vi "2100_Test_Set State_Measure Resistance_SH3T_Ron_w Config.vi"(0 "Semiconductor Module Context":T7, 1 "Script_Info":T3={"Script Name"="WalkingState", "All_Scripts"=[]}, 4 "Instrument_Pins":T6={"SMU_Pins"=["RF1", "RF2", "RF3", "RF4"], "HSDIO_Pins"=["CLK", "SDA"]}, 5 "Error In":errorcluster, 6 "USID":T4 max=15, 7 "Master_Register_Data_Array_In":T1 {"Address" format="%.0x"}, 8 "current range":dbl format="%#_6p", 9 "current level":dbl=1e-05 format="%#_13p", 10 "Publishable IDs":string[](array[string])=["State00", "State01", "State02", "State04", "State08"], 11 "Reg_Map_and_Bit_Name":T5={"Reg_Map_Bit_Name"="", "Reg_Map"=[["Reg Addr(0x00)", "7", "6", "5", "4", "3", "2", "1", "0"], ["0", "SPARE", "RF3_SH", "RF2_SH", "RF1_SH", "SPARE", "RF3_RFC", "RF2_RFC", "RF1_RFC"], ["1", "SPARE[7:0]", "", "", "", "", "", "", ""], ["2", "VVAR_EN", "LCM_EN", "RFC_SH", "SPARE", "VARACTOR[3:0]", "", "", ""], ["3", "SW_CTRL1_VIRTUAL[7:0]", "", "", "", "", "", "", ""], ["4", "SW_CTRL1_SWAP", "SW_CTRL1_RBSHIFT[2:0]", "", "", "SW_CTRL1_VSID[3:0]", "", "", ""], ["5", "REG_00_VIRTUAL_MASK[7:0]", "", "", "", "", "", "", ""], ["6", "LOCK_STATUS[1:0]", "", "CLK_DITHER", "FUSES_BURNED", "CLK_IDAC_CAL[3:0]", "", "", ""], ["7", "SPARE[2:0]", "", "", "ODFT_TRIM[4:0]", "", "", "", ""], ["8", "SPARE[2:0]", "", "", "HV_TRIM[4:0]", "", "", "", ""], ["9", "TEST_MUX[2:0]", "", "", "SPARE[1:0]", "", "MEMS_BG_TC[1:0]", "", "MEMSCP_RCM"], ["A", "CP_BOOST_OVRD_EN", "SPARE[2:0]", "", "", "PS_OFF_TIMER[1:0]", "", "PS_ON_TIMER[1:0]", ""], ["0", "", "", "", "", "", "", "", ""], ["D", "Reserved[1:0]", "", "WD_HI_EVENT_CNT[5:0]", "", "", "", "", ""], ["E", "VERSION_ID[7:0]", "", "", "", "", "", "", ""], ["F", "Reserved", "COUNT_200_LSB[6:0]", "", "", "", "", "", ""], ["10", "CLK_DIV2_EN", "Spare", "ODFT_EN", "HV_HYST[4:0]", "", "", "", ""], ["0", "", "", "", "", "", "", "", ""], ["12", "SHORT_FUSE", "FUSE_BURN", "STROBE_EN", "VIO_OK", "RTH[1:0]", "", "FUSE_LOAD_MAN_EN", "FUSE_LOAD"], ["13", "RR_ACK_EN", "Reserved", "ACK_POSITION[1:0]", "", "SuBUS_DRIVE_STRENGTH[3:0]", "", "", ""], ["14", "TM_IO_EN", "TM_IO_SEL", "SuBUS_OVS[1:0]", "", "Reserved[3:0]", "", "", ""], ["15", "Reserved[4:0]", "", "", "", "", "SuBUS_VERSION_PRESENT", "SuBUS_VOLTAGE", "SuBUS_FLAVOR_DEF"], ["16", "PROG_STROBE1_DUR[7:0]", "", "", "", "", "", "", ""], ["17", "PROG_STROBE0_DUR[7:0]", "", "", "", "", "", "", ""], ["18", "Reserved[2:0]", "", "", "EFUSE_SINGLE_ADDR_SEL[4:0]", "", "", "", ""], ["19", "POLL_ADR[4:0]", "", "", "", "", "POLL_BC[2:0]", "", ""], ["1A", "SOFTWARE_RESET", "Reserved[6:0]", "", "", "", "", "", ""], ["1B", "Reserved[7:0]", "", "", "", "", "", "", ""], ["1C", "PWR_MODE_1", "PWR_MODE_0", "TRIGGER_MASK[2:0]", "", "", "TRIGGER[2:0]", "", ""], ["1D", "PRODUCT_ID[7:0]", "", "", "", "", "", "", ""], ["1E", "MANUFACTURER_ID_LSB[7:0]", "", "", "", "", "", "", ""], ["1F", "MANUFACTURER_ID_MSB[3:0]", "", "", "", "USID[3:0]", "", "", ""]]}, 12 "R_Guardian":dbl[](array[numeric])) -> (15 "Master_Register_Data_Array_Out":T1 {"Address" format="%.0x"}, 19 "Error Out":errorcluster)   [LabVIEW 2013]
uses:
  Controls/USID.ctl
  <vilib>/NI_TestStand_SemiconductorModule/NI_TestStand_Semiconductor_Module.lvlibp/PinMap/General/SemiconductorModuleContext.ctl
  Controls/Master_Reg_Data_Array.ctl
  Controls/Reg_Address_Data.ctl
  <vilib>/NI_TestStand_SemiconductorModule/NI_TestStand_Semiconductor_Module.lvlibp/PinMap/General/Publish/PublishDataDoubleFunctionalTest.vi
  <vilib>/NI_TestStand_SemiconductorModule/NI_TestStand_Semiconductor_Module.lvlibp
panel:
  out "Publishable IDs 2":string[](array[string])=["State00", "State01", "State02", "State04", "State08"]
  out "Logged_Data":dbl[](array[numeric]) format="%#_6p"
  out "R_Measurements":dbl[](array[numeric]) format="%#_6p"
  in  "Tab Control":enum32{"Test Info", "Instrument Settings"}(tab)
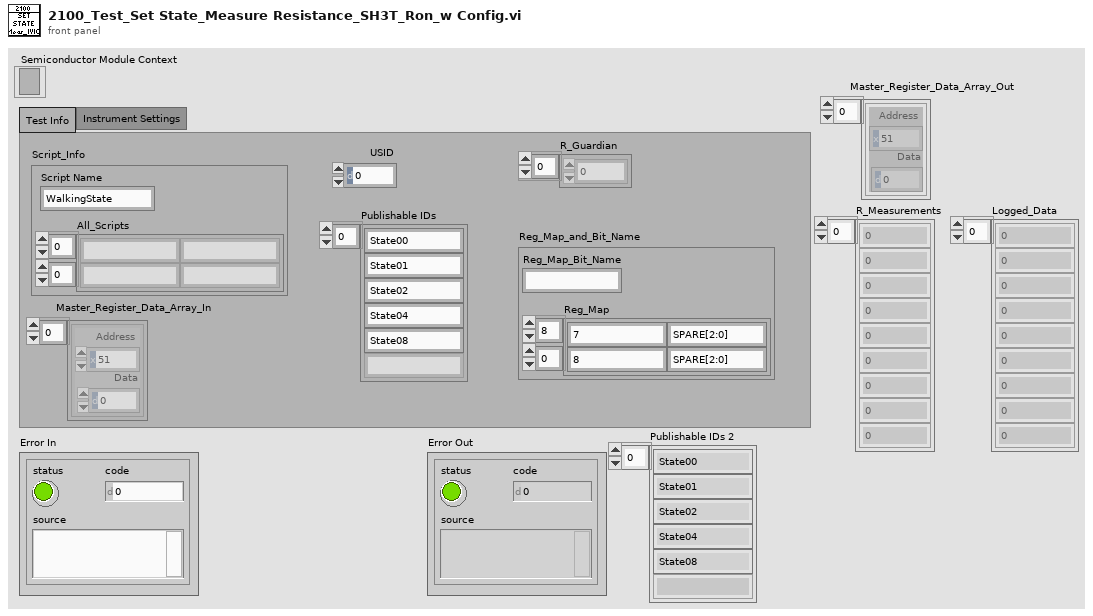
[diagram p1: front panel]
types:
  T1 = typedef "Master_Reg_Data_Array.ctl" = T2[]
  T2 = typedef "Reg_Address_Data.ctl" = cluster{"Address":u8, "Data":u8}
  T3 = cluster{"Script Name":string, "All_Scripts":string[][]}
  T4 = typedef "USID.ctl" = u8
  T5 = cluster{"Reg_Map_Bit_Name":string, "Reg_Map":string[][]}
  T6 = cluster{"SMU_Pins":string[], "HSDIO_Pins":string[]}
  T7 = typedef "NI_TestStand_Semiconductor_Module.lvlibp/SemiconductorModuleContext.ctl" = refnum<k7>
  T8 = typedef "Script Functions_Array.ctl" = enum16{"Reg_Write", "Bit_Write", "Delay", "Read", "Measure"}[]
  T9 = enum16{"Reg_Write", "Bit_Write", "Delay", "Read", "Measure"}
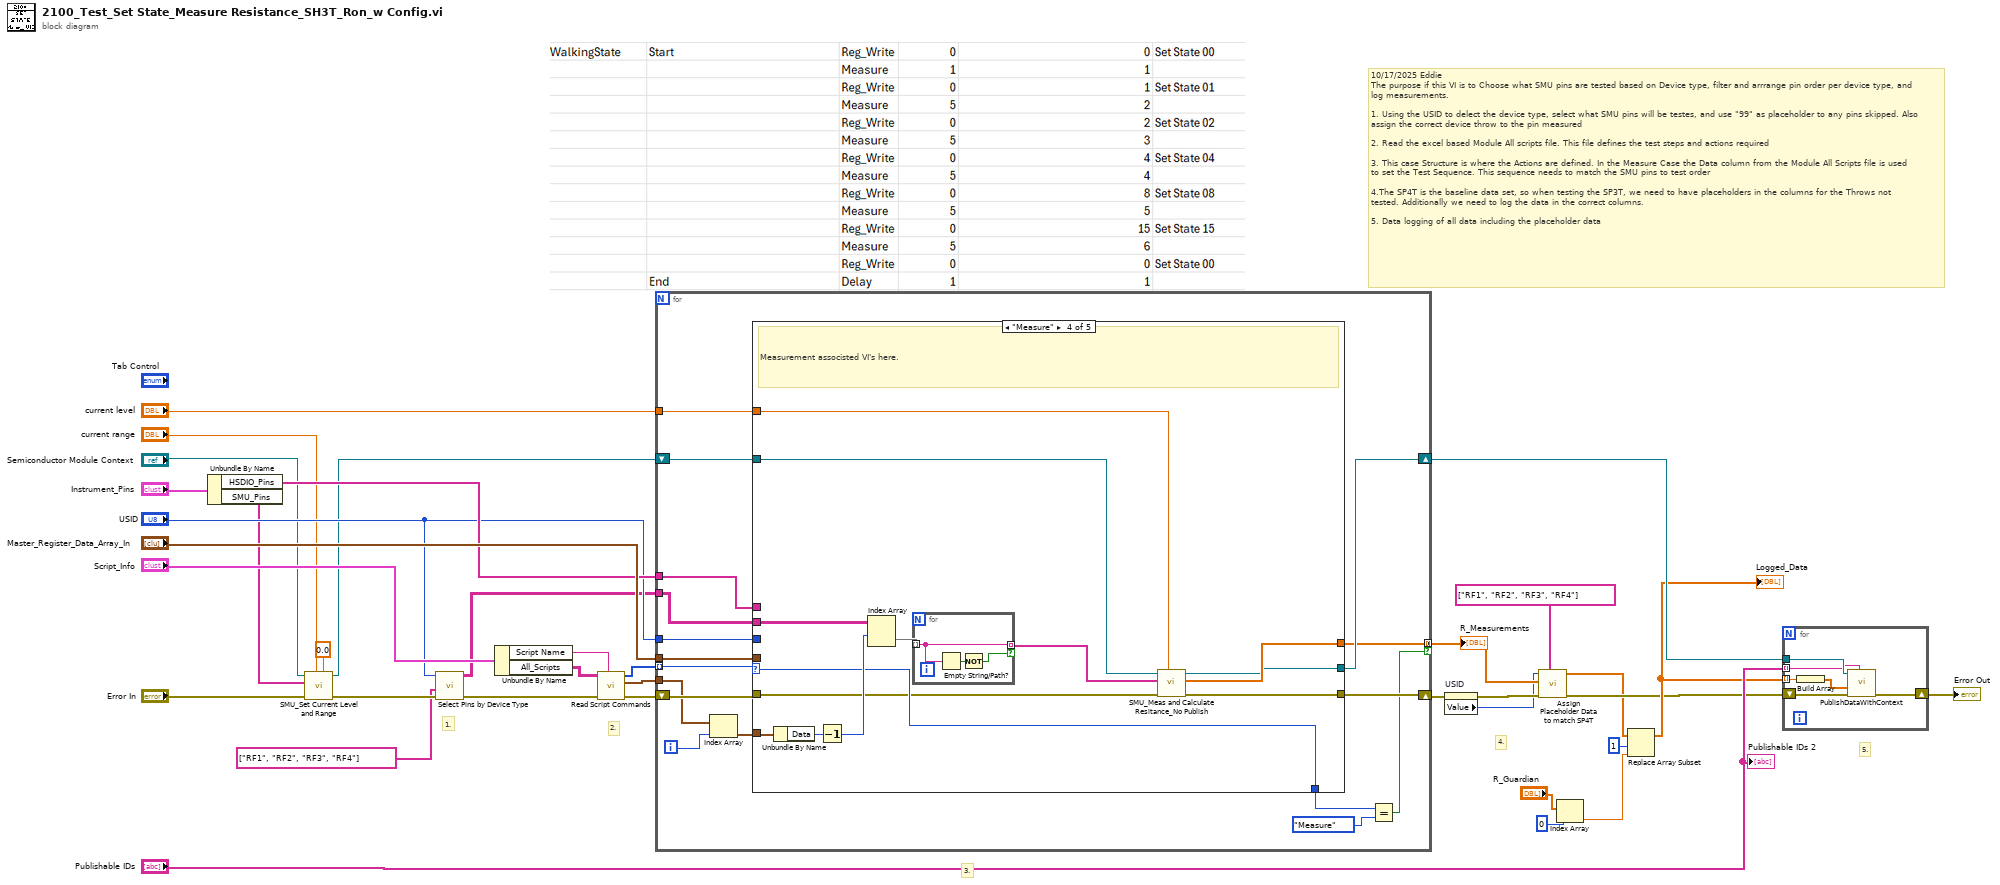
[diagram p0: block diagram]
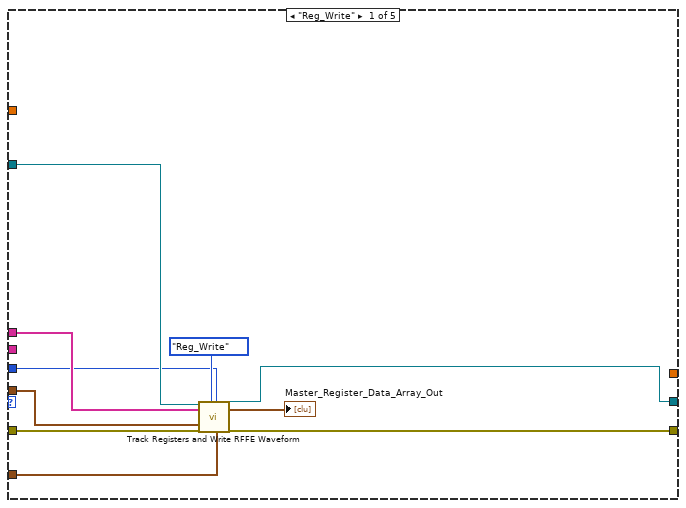
[diagram p2: hidden frame]
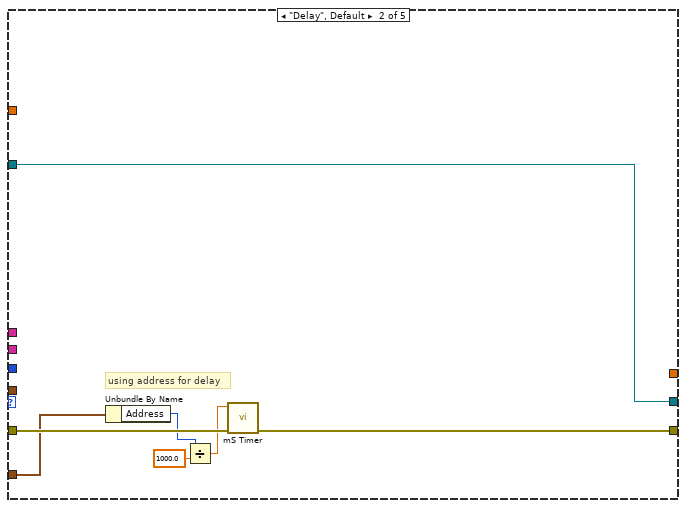
[diagram p3: hidden frame]
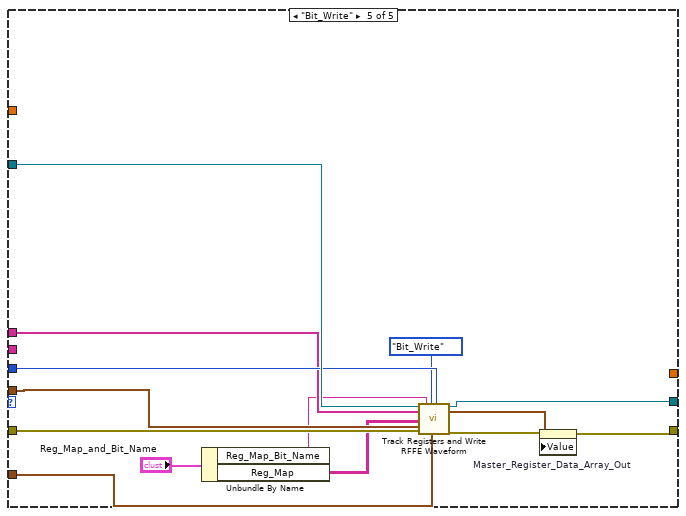
[diagram p5: hidden frame]
diagram:
  # "10/17/2025 Eddie \nThe purpose if this VI is to Choose what SMU pins are tested based on Device type, filter and arrrange pin order per device type, and log measurements.\n\n1. Using the USID to delect the device type, select what SMU pins will be testes, and use \"99\" as placeholder to any pins skipped. Also assign the correct device throw to the pin measured\n\n2. Read the excel based Module All scripts file. This file defines the test steps and actions required\n\n3. This case Structure is where the Actions are defined. In the Measure Case the Data column from the Module All Scripts file is used to set the Test Sequence. This sequence needs to match the SMU pins to test order\n\n4.The SP4T is the baseline data set, so when testing the SP3T, we need to have placeholders in the columns for the Throws not tested. Additionally we need to log the data in the correct columns.\n\n5. Data logging of all data including the placeholder data"
  # "5."
  # "4."
  # "3."
  # "2."
  # "1."
  n1 = Unbundle By Name("Instrument_Pins") -> ("HSDIO_Pins"=w31:string[], "SMU_Pins"=w5:string[])
  n2 = call "SMU_Set Current Level and Range.vi"("current level"=0.0, "current range"="current range", "error in (no error)"="Error In", "Pins"=w5, "Semiconductor Module Context"="Semiconductor Module Context") -> ("error out"=w8:errorcluster, "Semiconductor Module Context Out"=w6:T7)  [unwired: 5 in]
  n3 = call "Select Pins by Device Type.vi"("error in (no error)"=w8, "Publishable IDs"=string[] ["RF1", "RF2", "RF3", "RF4"] ("SP4T_Pins"), "USID"="USID") -> ("error out"=w27:errorcluster, "Pins to Test"=w25:string[][])  [unwired: 7 in]
  n4 = Unbundle By Name("Script_Info") -> ("Script Name"=w28:string, "All_Scripts"=w29:string[][])
  n5 = call "Read Script Commands.vi"("Test Name"=w28, "Error In"=w27, "All_Scripts"=w29) -> ("Error Out"=w34:errorcluster, "Script_Data"=w35:T2[], "Script_Functions"=w36:T8)  [unwired: 5 in, 1 out]
  n6 = for {
    tunnel: "USID" -> [w47]
    tunnel: w36 -> [w46] mode=indexing
    tunnel: w35 -> [w50]
    tunnel: w31 -> [w51]
    shift-right: [w44] -> w12
    shift-left: w34 -> [w53]
    tunnel: "Master_Register_Data_Array_In" -> [w48]
    tunnel: w25 -> [w43]
    shift-right: [w42] -> w23
    shift-left: w6 -> [w52]
    tunnel: [w41] -> w15 mode=concatenating if=w38
    tunnel: "current level" -> [w37]
    i -> [w45]
    n7 = Index Array(array=w50, index=w45) -> (element=w49:T2)
    n8 = case shown="\"Measure\"" w46 {
      selector: w46 -> [_ _ _ w80 _]
      tunnel: w49 -> [w58 w69 _ w85 w89]
      tunnel: w53 -> [w63 w70 w72 w79 w102]
      tunnel: w47 -> [w55 _ _ _ w96]
      tunnel: w52 -> [w61 w64 w71 w77 w97]
      tunnel: w51 -> [w60 _ _ _ w94]
      tunnel: [w62 w68 w72 w78 w100] -> w44
      tunnel: w48 -> [w57 _ _ _ w93]
      tunnel: w43 -> [_ _ _ w84 _]
      tunnel: [w54 w64 w71 w74 w98] -> w42
      tunnel: [_ _ _ w75 _] -> w41
      tunnel: [_ _ _ w80 _] -> w40
      tunnel: w37 -> [_ _ _ w73 _]
      frame "Reg_Write" {
        n9 = call "Track Registers and Write RFFE Waveform.vi"("Semiconductor Module Context"=w61, "Pins"=w60, "Master_Register_Data_Array_In"=w57, "Error In"=w63, "Script_Functions"=enum16{"Reg_Write", "Bit_Write"}."Reg_Write", "USID"=w55, "Reg_Address_Data"=w58) -> ("Semiconductor Module Context Out"=w54:T7, "Master_Register_Data_Array_Out"=→"Master_Register_Data_Array_Out":T1, "Error Out"=w62:errorcluster)  [unwired: 10 in]
      }
      frame "Delay", Default {
        # "using address for delay"
        n10 = Unbundle By Name(w69) -> ("Address"=w66:u8)
        n11 = Divide(x=w66, y=1000.0) -> (x/y=w65:dbl)
        n12 = call "mS Timer.vi"("Error In"=w70, "Delay(S)"=w65) -> ("Error Out"=w68:errorcluster)  [unwired: 9 in]
      }
      frame "Read" {
        # "Future Dev Code"
      }
      frame "Measure" {
        # "Measurement associsted VI's here."
        n13 = Unbundle By Name(w85) -> ("Data"=w82:u8)
        n14 = Decrement(x=w82) -> (x-1=w81:u8)
        n15 = Index Array(array=w84, index (row)=w81) -> (element=w83:string[])  [unwired: 1 in]
        n16 = for {
          tunnel: w83 -> [w88] mode=indexing
          tunnel: [w88] -> w76 mode=indexing if=w86
          n17 = Empty String/Path?(string/path=w88) -> (empty?=w87:bool)
          n18 = Not(x=w87) -> (.not. x?=w86:bool)
        }
        n19 = call "SMU_Meas and Calculate Resitance_No Publish.vi"("Current  Level"=w73, "error in (no error)"=w79, "Pins"=w76, "Semiconductor Module Context"=w77) -> ("error Out"=w78:errorcluster, "R Array"=w75:dbl[], "Semiconductor Module Context Out"=w74:T7)  [unwired: 4 in, 1 out]
      }
      frame "Bit_Write" {
        n20 = Unbundle By Name("Reg_Map_and_Bit_Name") -> ("Reg_Map_Bit_Name"=w91:string, "Reg_Map"=w90:string[][])
        n21 = call "Track Registers and Write RFFE Waveform.vi"("Semiconductor Module Context"=w97, "Pins"=w94, "Reg_Map"=w90, "Master_Register_Data_Array_In"=w93, "Error In"=w102, "Reg_Map_Bit_Name"=w91, "Script_Functions"=enum16{"Reg_Write", "Bit_Write"}."Bit_Write", "USID"=w96, "Reg_Address_Data"=w89) -> ("Semiconductor Module Context Out"=w98:T7, "Master_Register_Data_Array_Out"=w99:T1, "Error Out"=w101:errorcluster)  [unwired: 8 in]
        n22 = property on="Master_Register_Data_Array_Out" class="Arr (strict)"(error in=w101, "Value"=w99) -> (error out=w100:errorcluster)  [unwired: 1 in, 1 out]
      }
    }
    n23 = Equal?(x=w40, y=T9."Measure" ("Enum")) -> (x = y?=w38:bool)
  }
  "R_Measurements" <- w15
  n24 = property on="USID" class="DigNum (strict)"(error in=w12) -> (error out=w11:errorcluster, "Value"=w10:T4)  [unwired: 1 in, 1 out]
  n25 = call "Assign Placeholder Data to match SP4T.vi"("SP4T_Pins"=string[] ["RF1", "RF2", "RF3", "RF4"], "error in (no error)"=w11, "Individual_R_Meas"=w15, "USID"=w10) -> ("error out"=w17:errorcluster, "Placeholder_w_Data"=w14:dbl[])  [unwired: 6 in]
  n26 = Index Array(array="R_Guardian", index=0) -> (element=w18:dbl)
  n27 = Replace Array Subset(array=w14, new element=w18, index=1) -> (w19:dbl[])
  "Logged_Data" <- w19
  n28 = for {
    shift-right: [w108] -> w24
    shift-left: w17 -> [w107]
    tunnel: w23 -> [w106]
    tunnel: w19 -> [w105] mode=indexing
    tunnel: "Publishable IDs" -> [w103] mode=indexing
    n29 = Build Array(w105) -> (w104:dbl[])
    n30 = call-poly <vilib>:"PublishDataWithContext.vi"("Published Data Id"=w103, "error in (no error)"=w107, "Data In"=w104, "Semiconductor Module Context"=w106) -> ("error out"=w108:errorcluster)  [unwired: 6 in, 1 out]
  }
  "Error Out" <- w24
  "Publishable IDs 2" <- "Publishable IDs"
